vi "ProcessEvtTDC.vi"(8 "error in":errorcluster, 9 "Encoded Data":u32[](array[numeric]), 10 "# data points in evt":i32) -> (0 "error out":errorcluster, 1 "Decoded Data":cluster{"Channel":u8, "TDC Data":u16}[](array[cluster]), 2 "# Events":u32)   [LabVIEW 2014]
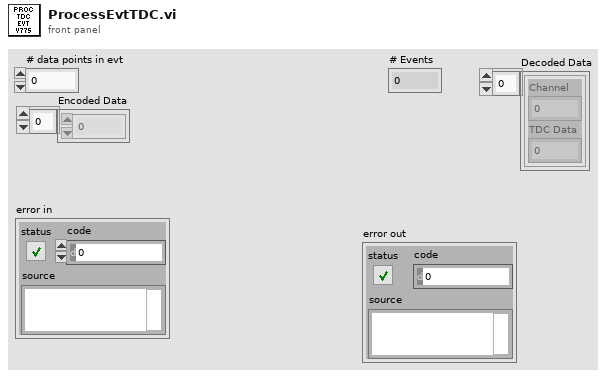
[diagram p1: front panel]
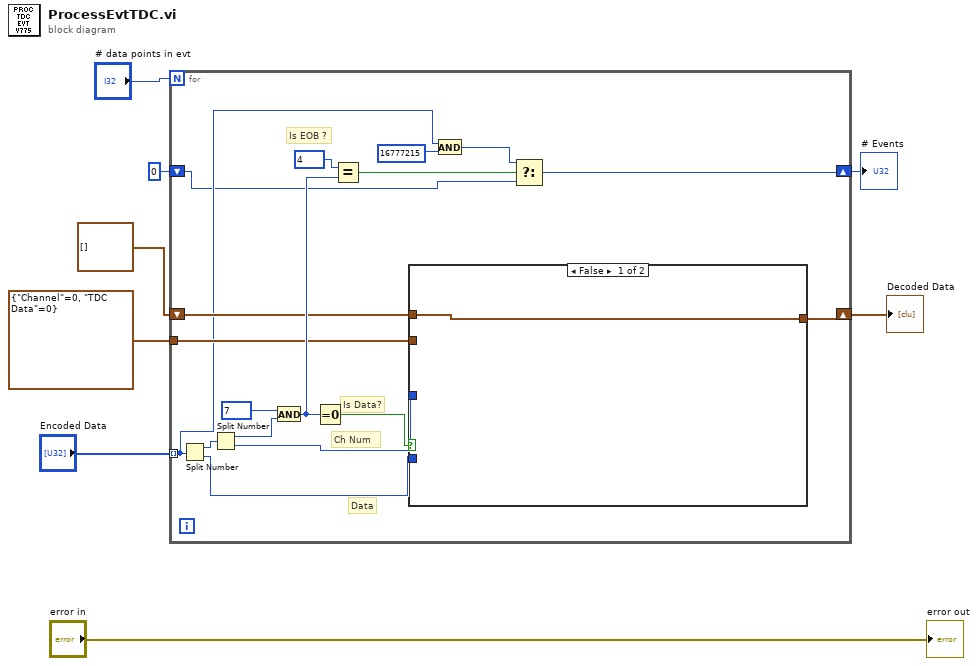
[diagram p0: block diagram]
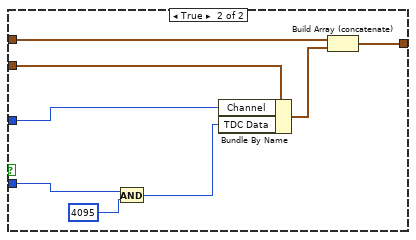
[diagram p2: hidden frame]
diagram:
  n1 = for {
    N: "# data points in evt" -> [_]
    tunnel: "Encoded Data" -> [w14] mode=indexing
    tunnel: cluster{"Channel":u8, "TDC Data":u16} {"Channel"=0, "TDC Data"=0} -> [w18]
    shift-right: [w10] -> w1
    shift-left: cluster{"Channel":u8, "TDC Data":u16}[] [] -> [w17]
    shift-right: [w12] -> w4
    shift-left: u32 0 -> [w11]
    # "Is EOB ?"
    # "Data"
    # "Is Data?"
    # "Ch Num"
    n2 = Split Number(x=w14) -> (hi(x)=w25:u16, lo(x)=w22:u16)
    n3 = Split Number(x=w25) -> (hi(x)=w23:u8, lo(x)=w9:u8)
    n4 = And(x=u8 7, y=w23) -> (x .and. y?=w19:u8)
    n5 = Equal To 0?(x=w19) -> (x = 0?=w21:bool)
    n6 = Equal?(x=u8 4, y=w19) -> (x = y?=w16:bool)
    n7 = case shown="False" w21 {
      tunnel: w22 -> [_ w33]
      tunnel: w9 -> [_ w31]
      tunnel: w18 -> [_ w32]
      tunnel: [w26 w29] -> w10
      tunnel: w17 -> [w26 w30]
      frame False {
      }
      frame True {
        n8 = And(x=w33, y=u16 4095) -> (x .and. y?=w27:u16)
        n9 = Bundle By Name(cluster=w32, "Channel"=w31, "TDC Data"=w27) -> (w28:cluster{"Channel":u8, "TDC Data":u16})
        n10 = Build Array (concatenate)(w30, w28) -> (w29:cluster{"Channel":u8, "TDC Data":u16}[])
      }
    }
    n11 = And(x=w14, y=u32 16777215 ("x")) -> (x .and. y?=w13:u32)
    n12 = Select(t=w13, s=w16, f=w11) -> (s? t:f=w12:u32)
  }
  "# Events" <- w4
  "Decoded Data" <- w1
  "error out" <- "error in"
